vi "Create.vi"(8 "ErrorIn":errorcluster, 9 "VIRef":refnum<vi>, 11 "ObjectIn":refnum<class "FrontPanelControl.lvclass">) -> (0 "ErrorOut":errorcluster, 3 "ObjectOut":refnum<class "FrontPanelControl.lvclass">)   [LabVIEW 2021, in "FrontPanelControl.lvclass"]
uses:
  FrontPanelControl.lvclass
  FrontPanelControl.lvclass/FrontPanelControl.ctl
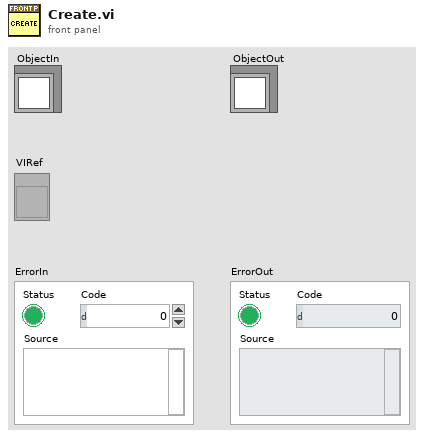
[diagram p1: front panel]
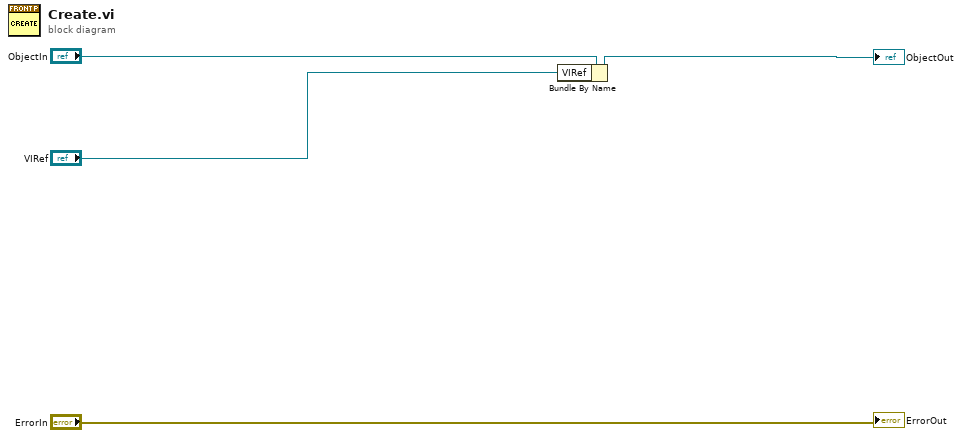
[diagram p0: block diagram]
diagram:
  n1 = Bundle By Name(cluster="ObjectIn", "VIRef"="VIRef") -> (→"ObjectOut":refnum<class "FrontPanelControl.lvclass">)
  "ErrorOut" <- "ErrorIn"
